vi "st_Binomial PDF (kx).vi"(9 "p":dbl=0.02, 10 "n":i32=100, 11 "x":dbl) -> (0 "error":i32, 3 "pdf(x)":dbl=0.13261955589475294)   [LabVIEW 2010, in "NI_Gmath.lvlib"]
uses:
  NI_Gmath.lvlib
  st_error_code.ctl
panel:
  # "Binomial PDF (kx)"
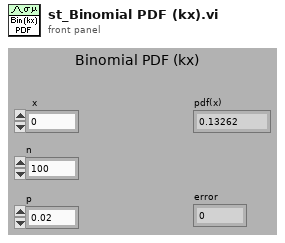
[diagram p1: front panel]
types:
  T1 = typedef "NI_Gmath.lvlib/st_error_code.ctl" = i32
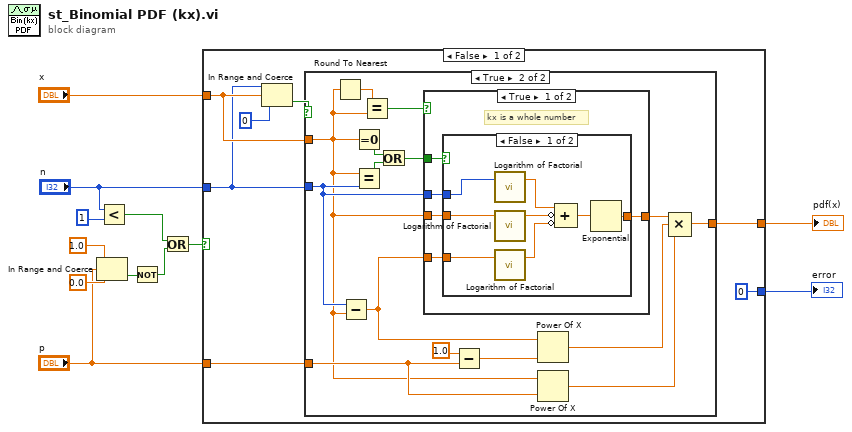
[diagram p0: block diagram]
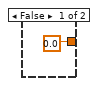
[diagram p2: hidden frame]
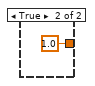
[diagram p3: hidden frame]
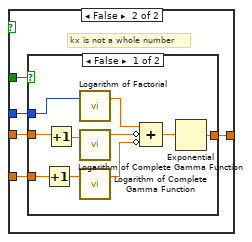
[diagram p4: hidden frame]
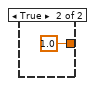
[diagram p5: hidden frame]
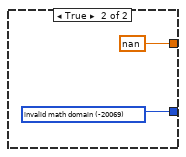
[diagram p6: hidden frame]
diagram:
  n1 = In Range and Coerce(upper limit=1.0, x="p", lower limit=0.0) -> (In Range?=w4:bool)  [unwired: 1 out]
  n2 = Less?(x="n", y=1) -> (x < y?=w2:bool)
  n3 = Not(x=w4) -> (.not. x?=w3:bool)
  n4 = Or(x=w2, y=w3) -> (x .or. y?=w7:bool)
  n5 = case shown="False" w7 {
    tunnel: [0 ("invalid math domain") w66] -> w12
    tunnel: [w14 nan] -> w11
    tunnel: "x" -> [w17 _]
    tunnel: "n" -> [w16 _]
    tunnel: "p" -> [w15 _]
    frame False {
      n6 = In Range and Coerce(upper limit=w16, x=w17, lower limit=0) -> (In Range?=w13:bool)  [unwired: 1 out]
      n7 = case shown="True" w13 {
        tunnel: [0.0 w28] -> w14
        tunnel: w17 -> [_ w23]
        tunnel: w16 -> [_ w24]
        tunnel: w15 -> [_ w32]
        frame False {
        }
        frame True {
          n8 = Round To Nearest(number=w23) -> (nearest integer value=w22:dbl)
          n9 = Subtract(x=w24, y=w23) -> (x-y=w27:dbl)
          n10 = Equal To 0?(x=w23) -> (x = 0?=w35:bool)
          n11 = Equal?(x=w23, y=w24) -> (x = y?=w34:bool)
          n12 = Equal?(x=w22, y=w23) -> (x = y?=w21:bool)
          n13 = Or(x=w35, y=w34) -> (x .or. y?=w25:bool)
          n14 = case shown="True" w21 {
            tunnel: w23 -> [w40 w54]
            tunnel: w27 -> [w39 w53]
            tunnel: [w38 w52] -> w26
            tunnel: w25 -> [w37 w51]
            tunnel: w24 -> [w36 w50]
            frame True {
              # "kx is a whole number"
              n15 = case shown="False" w37 {
                tunnel: w36 -> [w47 _]
                tunnel: w40 -> [w42 _]
                tunnel: w39 -> [w41 _]
                tunnel: [w45 1.0 ("t")] -> w38
                frame False {
                  n16 = call "Logarithm of Factorial.vi"("n"=w47) -> ("ln(n!)"=w48:dbl)  [unwired: 2 in]
                  n17 = call "Logarithm of Factorial.vi"("n"=w42) -> ("ln(n!)"=w44:dbl)  [unwired: 2 in]
                  n18 = call "Logarithm of Factorial.vi"("n"=w41) -> ("ln(n!)"=w43:dbl)  [unwired: 2 in]
                  n19 = Compound Arithmetic op=ADD(w48, invert w44, invert w43) -> (w46:dbl)
                  n20 = Exponential(1:w46) -> (0:w45:dbl)
                }
                frame True {
                }
              }
            }
            frame False {
              # "kx is not a whole number"
              n21 = case shown="False" w51 {
                tunnel: w50 -> [w63 _]
                tunnel: w54 -> [w60 _]
                tunnel: w53 -> [w57 _]
                tunnel: [w61 1.0 ("t")] -> w52
                frame False {
                  n22 = Increment(x=w57) -> (x+1=w56:dbl)
                  n23 = Increment(x=w60) -> (x+1=w59:dbl)
                  n24 = call "Logarithm of Factorial.vi"("n"=w63) -> ("ln(n!)"=w64:dbl)  [unwired: 2 in]
                  n25 = call "Logarithm of Complete Gamma Function.vi"("x"=w59) -> ("ln(g(x))"=w58:dbl)  [unwired: 2 in]
                  n26 = call "Logarithm of Complete Gamma Function.vi"("x"=w56) -> ("ln(g(x))"=w55:dbl)  [unwired: 2 in]
                  n27 = Compound Arithmetic op=ADD(w64, invert w58, invert w55) -> (w62:dbl)
                  n28 = Exponential(1:w62) -> (0:w61:dbl)
                }
                frame True {
                }
              }
            }
          }
          n29 = Subtract(x=1.0 ("t"), y=w32) -> (x-y=w33:dbl)
          n30 = Power Of X(1:w33, 2:w27) -> (0:w30:dbl)
          n31 = Power Of X(1:w32, 2:w23) -> (0:w29:dbl)
          n32 = Compound Arithmetic op=MULTIPLY(w26, w30, w29) -> (w28:dbl)
        }
      }
    }
    frame True {
      w66 = T1 -20069 items=["invalid math domain"=-20069, "Fourier interpolation size m >= n"=-20070, "empty array"=-20003] ("stat interp error code")
    }
  }
  "pdf(x)" <- w11
  "error" <- w12
